vi "FiletoDataHex (SubVI).vi"(8 "error constant":errorcluster, 10 "file path (use dialog)":path, 11 "Progress bar Max":refnum<vi>) -> (0 "error constant 2":errorcluster, 1 "Size of Text File":i32, 2 "Full Text File":u8[](array[numeric]) format="%.0x", 3 "All bytes in file in HEX U8":u8[](array[numeric]) format="%02x", 4 "Array 2":u8[](array[numeric]), 5 "Array":u8[](array[numeric]), 6 "sumHeader":u16 format="%.0x")   [LabVIEW 2017]
panel:
  out "Array 5":u8[][](array[numeric]) format="%02x"
  out "CheckSum DataB 2":u16 format="%.0x"
  out "conn ID":refnum<k5>
  in  "status":bool
  in  "Drv":u8(ring) items=["Drv 1", "Drv 2"]
  out "Writting Data":bool
  out "CheckSum Data":u16 format="%.0x"
  out "CheckSum DataB":u16 format="%.0x"
  # "0 TO 2053 = 2054 (2*1027)  CS = 77F0"
  # "2054 TO 4101 = 2048 (2*1024) CS = 4FF0"
  # "4102 TO 6149 = 2048 CS = 71DE"
  # "6150 TO 8197 = 2048 CS = 241D"
  # "8198 TO 10245 = 2048 CS = 404B"
  # "10246 TO 12293 = 2048 CS =  5235 --- 254E"
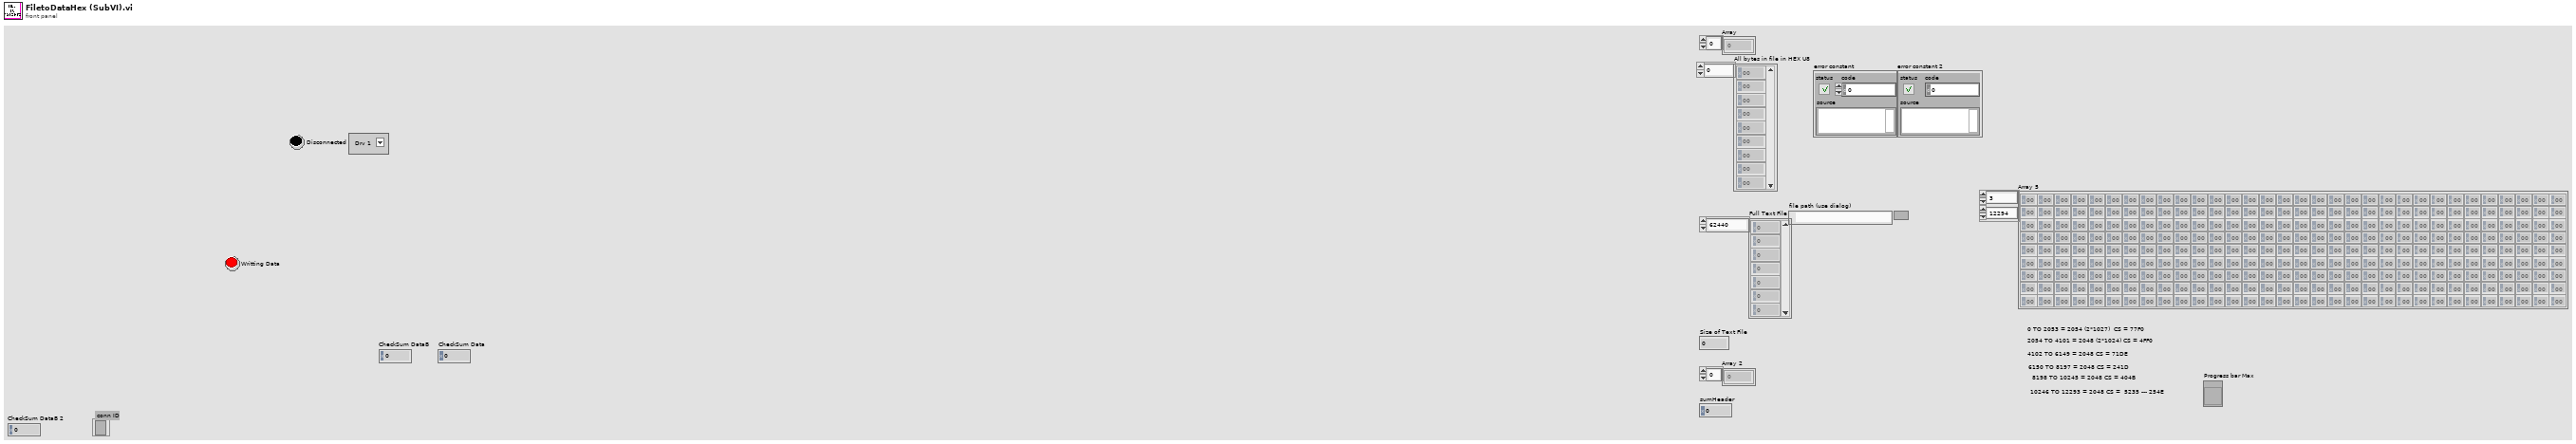
[diagram p1: front panel]
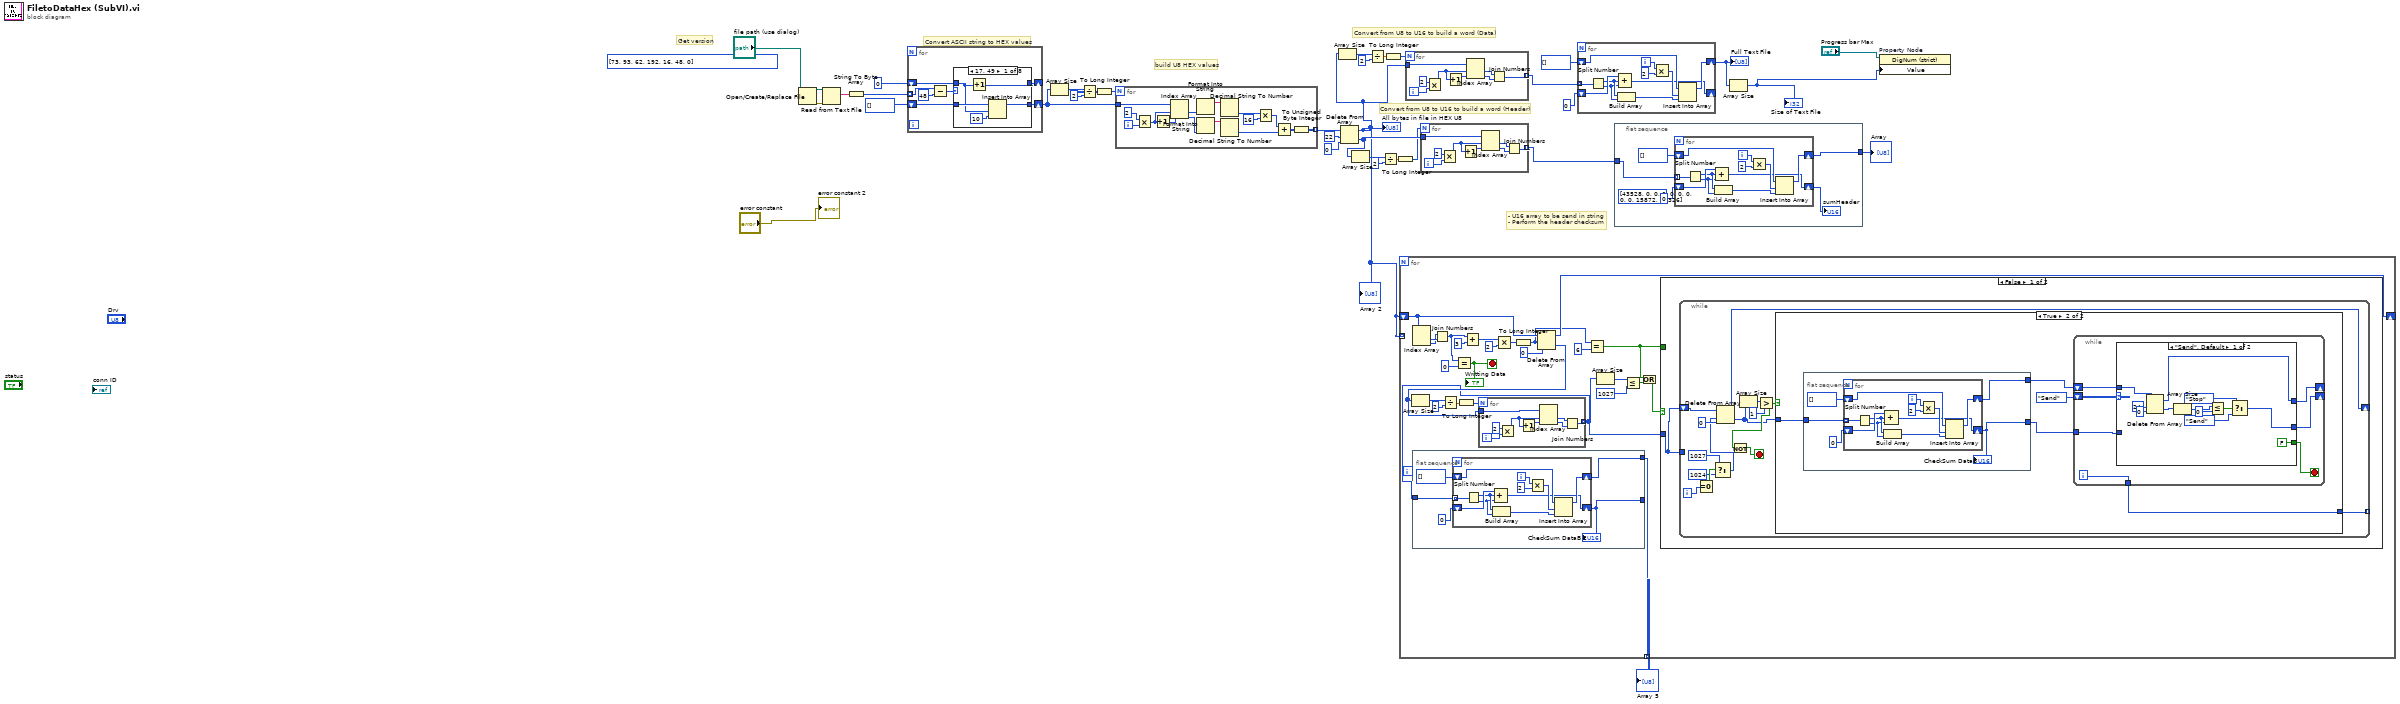
[diagram p0: block diagram]
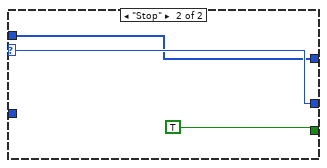
[diagram p3: hidden frame]
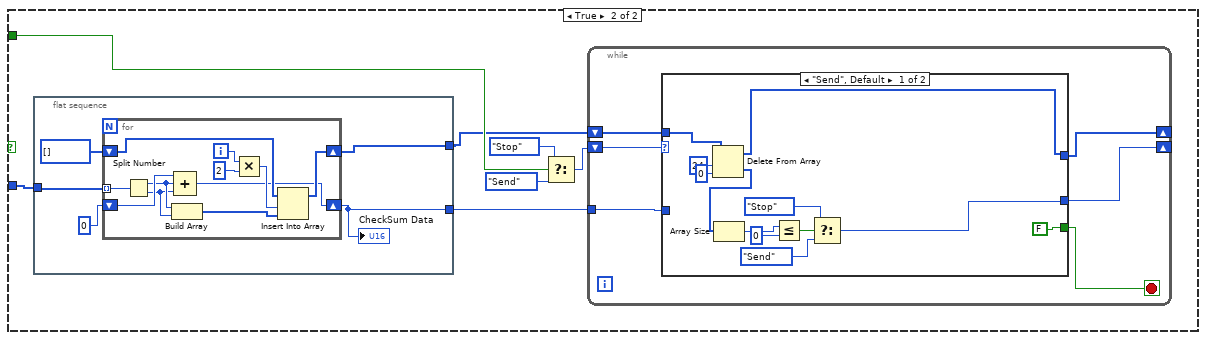
[diagram p4: hidden frame]
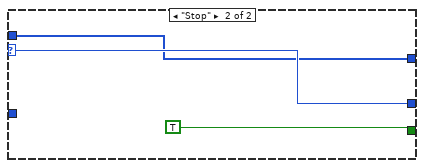
[diagram p5: hidden frame]
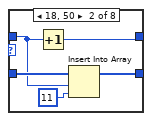
[diagram p6: hidden frame]
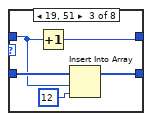
[diagram p7: hidden frame]
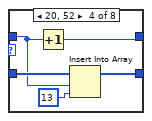
[diagram p8: hidden frame]
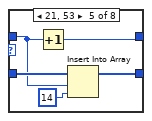
[diagram p9: hidden frame]
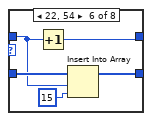
[diagram p10: hidden frame]
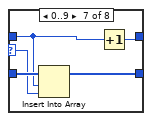
[diagram p11: hidden frame]
diagram:
  (unwired) u8[] [73, 93, 62, 192, 16, 48, 0] ("output array")
  # "Get version"
  # "- U16 array to be send in string\n- Perform the header checksum"
  # "Convert from U8 to U16 to build a word (Header)"
  # "build U8 HEX values"
  # "Convert from U8 to U16 to build a word (Data)"
  # "Convert ASCII string to HEX values"
  n1 = Open/Create/Replace File(file path (use dialog)="file path (use dialog)") -> (refnum out=w8:refnum<file>, error out=w7:errorcluster)  [unwired: 5 in, 1 out]
  n2 = Read from Text File(file (use dialog)=w8, error in=w7) -> (text=w10:string)  [unwired: 2 in, 3 out]
  n3 = String To Byte Array(string=w10) -> (unsigned byte array=w9:u8[])
  n4 = for {
    tunnel: w9 -> [w42] mode=indexing
    shift-right: [w38] -> w13
    shift-left: u8[] [] -> [w39]
    shift-right: [w37] -> _
    shift-left: 0 ("y") -> [w36]
    n5 = Subtract(x=w42, y=u8 48) -> (x-y=w40:u8)
    n6 = case shown="17, 49" w40 {
      selector: w40 -> [_ _ _ _ _ _ w76 _]
      tunnel: [w45 w50 w56 w60 w65 w70 w75 w79] -> w38
      tunnel: w39 -> [w47 w51 w57 w62 w67 w72 w77 w79]
      tunnel: [w43 w48 w53 w58 w63 w68 w73 w78] -> w37
      tunnel: w36 -> [w44 w49 w54 w59 w64 w69 w74 w78]
      frame 17, 49 {
        n7 = Increment(x=w44) -> (x+1=w43:i32)
        n8 = Insert Into Array(array=w47, index=w44, new element=u8 10) -> (w45:u8[])
      }
      frame 18, 50 {
        n9 = Increment(x=w49) -> (x+1=w48:i32)
        n10 = Insert Into Array(array=w51, index=w49, new element=u8 11) -> (w50:u8[])
      }
      frame 19, 51 {
        n11 = Increment(x=w54) -> (x+1=w53:i32)
        n12 = Insert Into Array(array=w57, index=w54, new element=u8 12) -> (w56:u8[])
      }
      frame 20, 52 {
        n13 = Increment(x=w59) -> (x+1=w58:i32)
        n14 = Insert Into Array(array=w62, index=w59, new element=u8 13) -> (w60:u8[])
      }
      frame 21, 53 {
        n15 = Increment(x=w64) -> (x+1=w63:i32)
        n16 = Insert Into Array(array=w67, index=w64, new element=u8 14) -> (w65:u8[])
      }
      frame 22, 54 {
        n17 = Increment(x=w69) -> (x+1=w68:i32)
        n18 = Insert Into Array(array=w72, index=w69, new element=u8 15) -> (w70:u8[])
      }
      frame 0..9 {
        n19 = Insert Into Array(array=w77, index=w74, new element=w76) -> (w75:u8[])
        n20 = Increment(x=w74) -> (x+1=w73:i32)
      }
      frame 240, Default {
      }
    }
  }
  n21 = Array Size(array=w13) -> (size(s)=w14:i32)
  n22 = Divide(x=w14, y=2) -> (x/y=w16:dbl)
  n23 = To Long Integer(number=w16) -> (32bit integer=w17:i32)
  n24 = for {
    N: w17 -> [_]
    tunnel: w13 -> [w94]
    tunnel: [w80] -> w18 mode=indexing
    i -> [w93]
    n25 = Multiply(x=2, y=w93) -> (x*y=w91:i32)
    n26 = Increment(x=w91) -> (x+1=w90:i32)
    n27 = Index Array(array=w94, index #1=w91, index #2=w90) -> (element #1=w83:u8, element #2=w82:u8)
    n28 = Format Into String(w83) -> (resulting string=w84:string)  [unwired: 3 in, 1 out]
    n29 = Format Into String(w82) -> (resulting string=w89:string)  [unwired: 3 in, 1 out]
    n30 = Decimal String To Number(string=w84) -> (number=w85:i32)  [unwired: 2 in, 1 out]
    n31 = Decimal String To Number(string=w89) -> (number=w88:i32)  [unwired: 2 in, 1 out]
    n32 = Multiply(x=w85, y=16) -> (x*y=w87:i32)
    n33 = Add(x=w87, y=w88) -> (x+y=w81:i32)
    n34 = To Unsigned Byte Integer(number=w81) -> (unsigned 8bit integer=w80:u8)
  }
  n35 = Delete From Array(array=w18, length=22, index=0) -> (deleted portion=w29:u8[], array with subset deleted=w4:u8[])
  "All bytes in file in HEX U8" <- w4
  "Array 2" <- w4
  n36 = Array Size(array=w4) -> (size(s)=w23:i32)
  n37 = Array Size(array=w29) -> (size(s)=w24:i32)
  n38 = Divide(x=w23, y=2) -> (x/y=w21:dbl)
  n39 = Divide(x=w24, y=2) -> (x/y=w26:dbl)
  n40 = To Long Integer(number=w21) -> (32bit integer=w28:i32)
  n41 = To Long Integer(number=w26) -> (32bit integer=w27:i32)
  n42 = for {
    shift-right: [w110] -> _
    shift-left: w4 -> [w120]
    tunnel: w4 -> [_] mode=indexing
    tunnel: [w95] -> w3 mode=indexing
    stop <- w113 stop-if-true
    n43 = Index Array(array=w120) -> (element #1=w119:u8, element #2=w118:u8)  [unwired: 2 in]
    n44 = flat-sequence {
      tunnel: [w123] -> w95
      tunnel: [w121] -> _
      tunnel: w96 -> [w122]
      frame #0 {
        n45 = for {
          tunnel: w122 -> [w136] mode=indexing
          shift-right: [w131] -> w123
          shift-left: u8[] [] -> [w130]
          shift-right: [w128] -> w121
          shift-left: u16 0 -> [w129]
          i -> [w135]
          n46 = Split Number(x=w136) -> (hi(x)=w127:u8, lo(x)=w126:u8)
          n47 = Build Array(w127, w126) -> (w133:u8[])
          n48 = Compound Arithmetic op=ADD(w129, w127, w126) -> (w128:u16)
          n49 = Multiply(x=w135, y=2) -> (x*y=w132:i32)
          n50 = Insert Into Array(array=w130, index=w132, new element=w133) -> (w131:u8[])
        }
        "CheckSum DataB 2" <- w121
      }
    }
    n51 = Join Numbers(hi=w118, lo=w119) -> ((hi.lo)=w98:u16)
    n52 = Equal?(x=w98, y=u16 0) -> (x = y?=w113:bool)
    "Writting Data" <- w113
    n53 = Add(x=w98, y=u32 3) -> (x+y=w116:u32)
    n54 = Multiply(x=w116, y=u32 2) -> (x*y=w114:u32)
    n55 = To Long Integer(number=w114) -> (32bit integer=w99:i32)
    n56 = Delete From Array(array=w120, length=w99, index=0) -> (deleted portion=w100:u8[], array with subset deleted=w110:u8[])
    n57 = Array Size(array=w100) -> (size(s)=w107:i32)
    n58 = Divide(x=w107, y=2) -> (x/y=w109:dbl)
    n59 = To Long Integer(number=w109) -> (32bit integer=w106:i32)
    n60 = for {
      N: w106 -> [_]
      tunnel: w100 -> [w243]
      tunnel: [w239] -> w96 mode=indexing
      i -> [w242]
      n61 = Multiply(x=2, y=w242) -> (x*y=w245:i32)
      n62 = Increment(x=w245) -> (x+1=w246:i32)
      n63 = Index Array(array=w243, index #1=w245, index #2=w246) -> (element #1=w241:u8, element #2=w240:u8)
      n64 = Join Numbers(hi=w241, lo=w240) -> ((hi.lo)=w239:u16)
    }
    n65 = Equal?(x=w99, y=6) -> (x = y?=w97:bool)
    n66 = Array Size(array=w96) -> (size(s)=w105:i32)
    n67 = Less Or Equal?(x=w105, y=1027) -> (x <= y?=w102:bool)
    n68 = Or(x=w97, y=w102) -> (x .or. y?=w101:bool)
    n69 = case shown="False" w101 {
      tunnel: w96 -> [w137 w201]
      tunnel: w97 -> [_ w197]
      frame False {
        n70 = while {
          tunnel: w137 -> [_]
          shift-right: [w144] -> _
          shift-left: w137 -> [w151]
          tunnel: [w138] -> _ mode=indexing
          i -> [w143]
          stop <- w146 stop-if-true
          n71 = Equal To 0?(x=w143) -> (x = 0?=w142:bool)
          n72 = Select(t=1027 ("length"), s=w142, f=1024 ("length")) -> (s? t:f=w139:i32)
          n73 = Delete From Array(array=w151, length=w139, index=0) -> (deleted portion=w145:u16[], array with subset deleted=w144:u16[])
          n74 = Array Size(array=w145) -> (size(s)=w149:i32)
          n75 = Greater?(x=w149, y=1) -> (0:w147:bool)
          n76 = Not(x=w147) -> (.not. x?=w146:bool)
          n77 = case shown="True" w147 {
            tunnel: w145 -> [_ w156]
            tunnel: [_ w153] -> w138
            frame False {
            }
            frame True {
              n78 = flat-sequence {
                tunnel: [w181] -> w152
                tunnel: [w179] -> w154
                tunnel: w156 -> [w180]
                frame #0 {
                  n79 = for {
                    tunnel: w180 -> [w194] mode=indexing
                    shift-right: [w189] -> w181
                    shift-left: u8[] [] -> [w188]
                    shift-right: [w186] -> w179
                    shift-left: u16 0 -> [w187]
                    i -> [w193]
                    n80 = Split Number(x=w194) -> (hi(x)=w185:u8, lo(x)=w184:u8)
                    n81 = Build Array(w185, w184) -> (w191:u8[])
                    n82 = Compound Arithmetic op=ADD(w187, w185, w184) -> (w186:u16)
                    n83 = Multiply(x=w193, y=2) -> (x*y=w190:i32)
                    n84 = Insert Into Array(array=w188, index=w190, new element=w191) -> (w189:u8[])
                  }
                  "CheckSum DataB" <- w179
                }
              }
              n85 = while {
                shift-right: [w161] -> _
                shift-left: enum16{"Stop", "Receive", "Send"}."Send" -> [w163]
                shift-right: [w159] -> _
                shift-left: w152 -> [w162]
                tunnel: w154 -> [w160]
                tunnel: [w158] -> w153
                i -> [w158]
                stop <- w157 stop-if-true
                n86 = case shown="\"Send\", Default" w163 {
                  selector: w163 -> [_ w178]
                  tunnel: w162 -> [w173 w176]
                  tunnel: [w170 w178] -> w161
                  tunnel: w160 -> [_ _]
                  tunnel: [FALSE TRUE] -> w157
                  tunnel: [w166 w176] -> w159
                  frame "Send", Default {
                    n87 = Delete From Array(array=w173, length=24, index=0) -> (deleted portion=w165:u8[], array with subset deleted=w166:u8[])
                    n88 = Array Size(array=w165) -> (size(s)=w171:i32)
                    n89 = Less Or Equal?(x=w171, y=0) -> (x <= y?=w164:bool)
                    n90 = Select(t=enum16{"Stop", "Receive", "Send"}."Stop", s=w164, f=enum16{"Stop", "Receive", "Send"}."Send") -> (s? t:f=w170:enum16{"Stop", "Receive", "Send"})
                  }
                  frame "Stop" {
                  }
                }
              }
            }
          }
        }
      }
      frame True {
        n91 = flat-sequence {
          tunnel: [w225] -> w195
          tunnel: w201 -> [w224]
          tunnel: [w223] -> w200
          frame #0 {
            n92 = for {
              tunnel: w224 -> [w238] mode=indexing
              shift-right: [w233] -> w225
              shift-left: u8[] [] -> [w232]
              shift-right: [w230] -> w223
              shift-left: u16 0 -> [w231]
              i -> [w237]
              n93 = Split Number(x=w238) -> (hi(x)=w229:u8, lo(x)=w228:u8)
              n94 = Build Array(w229, w228) -> (w235:u8[])
              n95 = Compound Arithmetic op=ADD(w231, w229, w228) -> (w230:u16)
              n96 = Multiply(x=w237, y=2) -> (x*y=w234:i32)
              n97 = Insert Into Array(array=w232, index=w234, new element=w235) -> (w233:u8[])
            }
            "CheckSum Data" <- w223
          }
        }
        n98 = Select(t=enum16{"Stop", "Receive", "Send"}."Stop", s=w197, f=enum16{"Stop", "Receive", "Send"}."Send") -> (s? t:f=w198:enum16{"Stop", "Receive", "Send"})
        n99 = while {
          shift-right: [w205] -> _
          shift-left: w198 -> [w207]
          shift-right: [w203] -> _
          shift-left: w195 -> [w206]
          tunnel: w200 -> [w204]
          stop <- w202 stop-if-true
          n100 = case shown="\"Send\", Default" w207 {
            selector: w207 -> [_ w222]
            tunnel: w206 -> [w217 w220]
            tunnel: [w214 w222] -> w205
            tunnel: w204 -> [_ _]
            tunnel: [FALSE TRUE] -> w202
            tunnel: [w210 w220] -> w203
            frame "Send", Default {
              n101 = Delete From Array(array=w217, length=24, index=0) -> (deleted portion=w208:u8[], array with subset deleted=w210:u8[])
              n102 = Array Size(array=w208) -> (size(s)=w215:i32)
              n103 = Less Or Equal?(x=w215, y=0) -> (x <= y?=w209:bool)
              n104 = Select(t=enum16{"Stop", "Receive", "Send"}."Stop", s=w209, f=enum16{"Stop", "Receive", "Send"}."Send") -> (s? t:f=w214:enum16{"Stop", "Receive", "Send"})
            }
            frame "Stop" {
            }
          }
        }
      }
    }
  }
  "Array 5" <- w3
  n105 = for {
    N: w28 -> [_]
    tunnel: w4 -> [w251]
    tunnel: [w247] -> w34 mode=indexing
    i -> [w250]
    n106 = Multiply(x=2, y=w250) -> (x*y=w253:i32)
    n107 = Increment(x=w253) -> (x+1=w254:i32)
    n108 = Index Array(array=w251, index #1=w253, index #2=w254) -> (element #1=w249:u8, element #2=w248:u8)
    n109 = Join Numbers(hi=w249, lo=w248) -> ((hi.lo)=w247:u16)
  }
  n110 = for {
    N: w27 -> [_]
    tunnel: w29 -> [w259]
    tunnel: [w255] -> w30 mode=indexing
    i -> [w258]
    n111 = Multiply(x=2, y=w258) -> (x*y=w261:i32)
    n112 = Increment(x=w261) -> (x+1=w262:i32)
    n113 = Index Array(array=w259, index #1=w261, index #2=w262) -> (element #1=w257:u8, element #2=w256:u8)
    n114 = Join Numbers(hi=w257, lo=w256) -> ((hi.lo)=w255:u16)
  }
  n115 = for {
    tunnel: w34 -> [w273] mode=indexing
    shift-right: [w268] -> w33
    shift-left: u8[] [] -> [w267]
    shift-right: [w265] -> _
    shift-left: u16 0 -> [w266]
    i -> [w272]
    n116 = Split Number(x=w273) -> (hi(x)=w264:u8, lo(x)=w263:u8)
    n117 = Build Array(w264, w263) -> (w270:u8[])
    n118 = Compound Arithmetic op=ADD(w266, w264, w263) -> (w265:u16)
    n119 = Multiply(x=w272, y=2) -> (x*y=w269:i32)
    n120 = Insert Into Array(array=w267, index=w269, new element=w270) -> (w268:u8[])
  }
  "Full Text File" <- w33
  n121 = flat-sequence {
    tunnel: [w276] -> w35
    tunnel: w30 -> [w275]
    frame #0 {
      (unwired) u16[] [43528, 0, 0, 0, 0, 0, 0, 0, 0, 15872, 36326]
      n122 = for {
        tunnel: w275 -> [w289] mode=indexing
        shift-right: [w284] -> w276
        shift-left: u8[] [] -> [w283]
        shift-right: [w281] -> w274
        shift-left: u16 0 -> [w282]
        i -> [w288]
        n123 = Split Number(x=w289) -> (hi(x)=w280:u8, lo(x)=w279:u8)
        n124 = Build Array(w280, w279) -> (w286:u8[])
        n125 = Compound Arithmetic op=ADD(w282, w280, w279) -> (w281:u16)
        n126 = Multiply(x=w288, y=2) -> (x*y=w285:i32)
        n127 = Insert Into Array(array=w283, index=w285, new element=w286) -> (w284:u8[])
      }
      "sumHeader" <- w274
    }
  }
  n128 = Array Size(array=w33) -> (size(s)=w1:i32)
  "Size of Text File" <- w1
  n129 = property on="Property Node" class="DigNum (strict)"(reference="Progress bar Max", "Value"=w1) -> ()  [unwired: 1 in, 2 out]
  "Array" <- w35
  "error constant 2" <- "error constant"
